vi "Returning Values By Reference 2D Array Of Integers.vi"(8 "error in (no error)":errorcluster, 9 "newArray":i32, 10 "cols":i32, 11 "rows":i32) -> (0 "error out":errorcluster, 1 "newArray out":i32)   [LabVIEW 2009, in "LabVIEWWrapper_PassingDataSampleDLL.lvlib"]
doc: "void ReturningValuesByReference_2DArrayOfIntegers (int rows, int cols, int ***newArray);"
uses:
  LabVIEWWrapper_PassingDataSampleDLL.lvlib
  PassingDataSampleDLL.dll
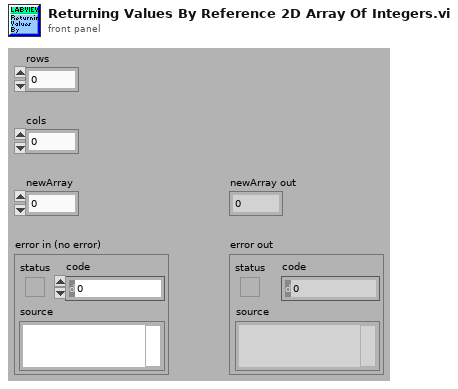
[diagram p1: front panel]
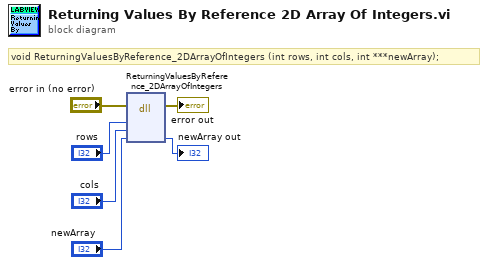
[diagram p0: block diagram]
diagram:
  # "void ReturningValuesByReference_2DArrayOfIntegers (int rows, int cols, int ***newArray);"
  n1 = dll-call lib="C:/My Dropbox/Systems Engineering Application/SDK/C Integration/LabVIEWWrapper/PassingDataSampleDLL.*" fn="ReturningValuesByReference_2DArrayOfIntegers"(error in="error in (no error)", "rows"="rows", "cols"="cols", "newArray"="newArray") -> (error out=→"error out":errorcluster, "newArray"=→"newArray out":i32)  [unwired: 5 in, 1 out]
